vi "example_dll.vi"(8 "Error In":errorcluster) -> (0 "Error Out":errorcluster)   [LabVIEW 2014]
panel:
  out "b":i32
  in  "a":i32
  out "numout":i32[](array[numeric])
  in  "Array":i32[](array[numeric])
  in  "Array 2":i32[](array[numeric])
  out "number out 2":i32
  in  "number in":i32
  out "number out":i32
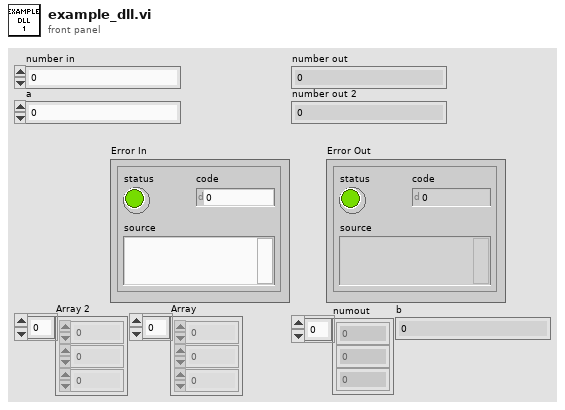
[diagram p1: front panel]
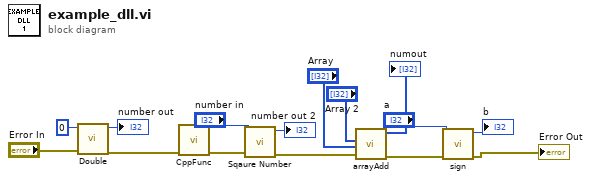
[diagram p0: block diagram]
diagram:
  n1 = call "Double.vi"("Error In"="Error In", "number in"=0) -> ("Error Out"=w12:errorcluster, "number out"=→"number out":i32)  [unwired: 8 in]
  n2 = call "CppFunc.vi"("Error In"=w12) -> ("Error Out"=w11:errorcluster)  [unwired: 10 in]
  n3 = call "Sqaure Number.vi"("Error In"=w11, "number in"="number in") -> ("Error Out"=w8:errorcluster, "number out"=→"number out 2":i32)  [unwired: 8 in]
  n4 = call "arrayAdd.vi"("error in"=w8, "Array2"="Array 2", "Array"="Array") -> ("error out"=w4:errorcluster, "numberOut"=→"numout":i32[])  [unwired: 7 in]
  n5 = call "sign.vi"("Error In"=w4, "number in"="a") -> ("Error Out"=→"Error Out":errorcluster, "number out"=→"b":i32)  [unwired: 8 in]
